vi "ROI转换.vi"(0 "左上x轴+":i32, 1 "左上y轴+":i32, 2 "右下x轴-":i32, 3 "右下y轴-":i32, 4 "ROI输入(T3)":T1) -> (5 "ROI输出(T2)":T1)   [LabVIEW 2017]
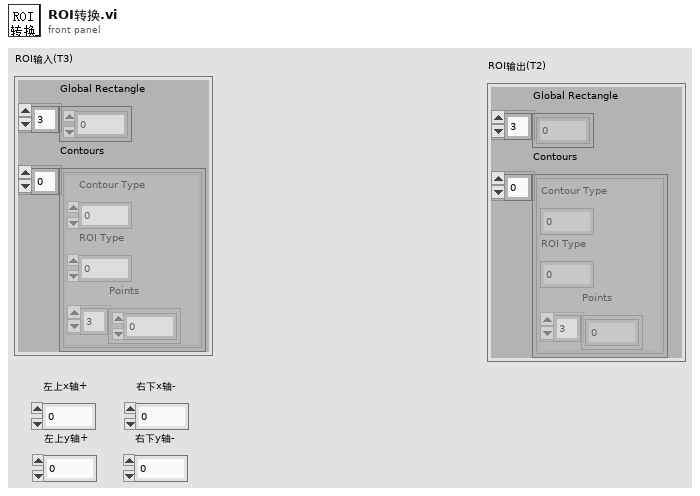
[diagram p1: front panel]
types:
  T1 = cluster{"Global Rectangle":i32[], "Contours":cluster{"Contour Type":u32, "ROI Type":u32, "Points":i32[]}[]}
  T2 = cluster{"Contour Type":u32, "ROI Type":u32, "Points":i32[]}[]
  T3 = cluster{"Contour Type":u32, "ROI Type":u32, "Points":i32[]}
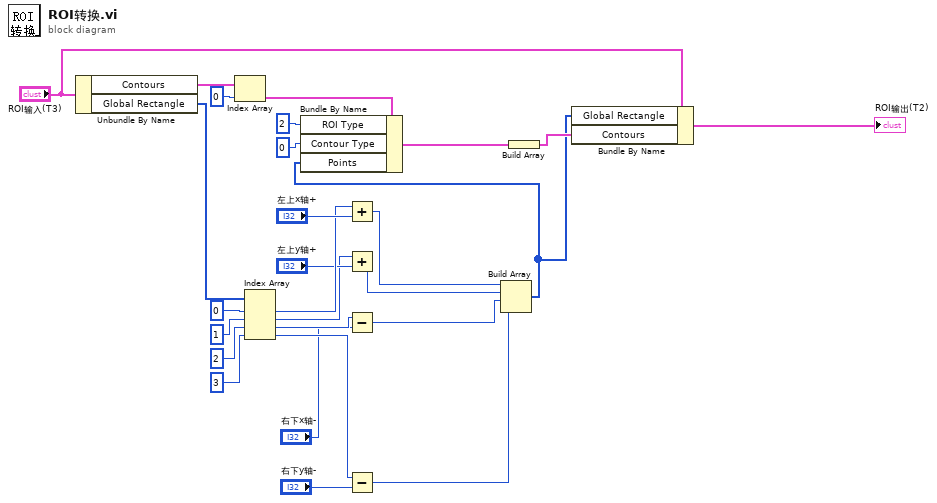
[diagram p0: block diagram]
diagram:
  n1 = Unbundle By Name("ROI输入(T3)") -> ("Contours"=w27:T2, "Global Rectangle"=w22:i32[])
  n2 = Index Array(array=w27, index=0 ("索引")) -> (element=w25:T3)
  n3 = Index Array(array=w22, index #1=u32 0 ("ROI Type"), index #2=u32 1 ("ROI Type"), index #3=u32 2 ("ROI Type"), index #4=u32 3 ("ROI Type")) -> (element #1=w16:i32, element #2=w14:i32, element #3=w2:i32, element #4=w13:i32)
  n4 = Add(x=w16, y="左上x轴+") -> (x+y=w11:i32)
  n5 = Add(x=w14, y="左上y轴+") -> (x+y=w10:i32)
  n6 = Subtract(x=w2, y="右下x轴-") -> (x-y=w9:i32)
  n7 = Subtract(x=w13, y="右下y轴-") -> (x-y=w8:i32)
  n8 = Build Array(w11, w10, w9, w8) -> (w4:i32[])
  n9 = Bundle By Name(cluster=w25, "ROI Type"=u32 2, "Contour Type"=u32 0 ("ROI Type"), "Points"=w4) -> (w7:T3)
  n10 = Build Array(w7) -> (w5:T2)
  n11 = Bundle By Name(cluster="ROI输入(T3)", "Global Rectangle"=w4, "Contours"=w5) -> (→"ROI输出(T2)":T1)
